vi "FPGA_DATA.vi"() -> ()   [LabVIEW 2019]
uses:
  <vilib>/LabVIEW Targets/FPGA/RIO/nicrio_985x_controls.llb/CAN_IO_Frame Cluster.ctl
  <vilib>/LabVIEW Targets/FPGA/RIO/nicrio_985x_controls.llb/CAN_IO_Frame Type.ctl
  <vilib>/rvi/Emulation/niFpgaGetClockAttributes.vi
  <vilib>/rvi/Emulation/niFpgaSctlEmulationGetInTimedLoop.vi
  <vilib>/rvi/Emulation/niFpgaEmulationReportErrorSimple.vi
  <vilib>/rvi/eio/common/nirviEmuTemplateMethod_errors.vi
  <vilib>/rvi/Emulation/niFpgaCriticalErrorInLSC.vi
  <vilib>/eio/EIONode/EIONode.xnode
panel:
  in  "DIO1":bool
  in  "CAN1 write":T1={"배열[0]"={"timestamp high"=0, "timestamp low"=0, "identifier"=0, "type"=enum."Data Frame", "info A"=0, "info B"=0, "data length"=0, "data"=[0, 0, 0, 0, 0, 0, 0, 0]}, "배열[1]"={"timestamp high"=0, "timestamp low"=0, "identifier"=0, "type"=enum."Data Frame", "info A"=0, "info B"=0, "data length"=0, "data"=[0, 0, 0, 0, 0, 0, 0, 0]}, "배열[2]"={"timestamp high"=0, "timestamp low"=0, "identifier"=0, "type"=enum."Data Frame", "info A"=0, "info B"=0, "data length"=0, "data"=[0, 0, 0, 0, 0, 0, 0, 0]}, "배열[3]"={"timestamp high"=0, "timestamp low"=0, "identifier"=0, "type"=enum."Data Frame", "info A"=0, "info B"=0, "data length"=0, "data"=[0, 0, 0, 0, 0, 0, 0, 0]}, "배열[4]"={"timestamp high"=0, "timestamp low"=0, "identifier"=0, "type"=enum."Data Frame", "info A"=0, "info B"=0, "data length"=0, "data"=[0, 0, 0, 0, 0, 0, 0, 0]}}
  out "L_force":sgl
  out "R_force":sgl
  out "CAN1 read":T2={"배열 2[0]"={"timestamp high"=0, "timestamp low"=0, "identifier"=0, "type"=enum."Data Frame", "info A"=0, "info B"=0, "data length"=0, "data"=[0, 0, 0, 0, 0, 0, 0, 0]}}
  in  "Write_que":bool
  out "Mod1/CAN1":T3={"timestamp high"=0, "timestamp low"=0, "identifier"=0, "type"=enum."Data Frame", "info A"=0, "info B"=0, "data length"=0, "data"=[0, 0, 0, 0, 0, 0, 0, 0]} {"identifier" format="%x"; "timestamp high" format="%08x"; "timestamp low" format="%08x"; "data" format="%.0x"}
  in  "D2":bool
  out "IMUS":sgl[](array[numeric])
  out "Mod1/CAN0":T3={"timestamp high"=0, "timestamp low"=0, "identifier"=0, "type"=enum."Data Frame", "info A"=0, "info B"=0, "data length"=0, "data"=[0, 0, 0, 0, 0, 0, 0, 0]} {"identifier" format="%x"; "timestamp high" format="%08x"; "timestamp low" format="%08x"; "data" format="%.0x"}
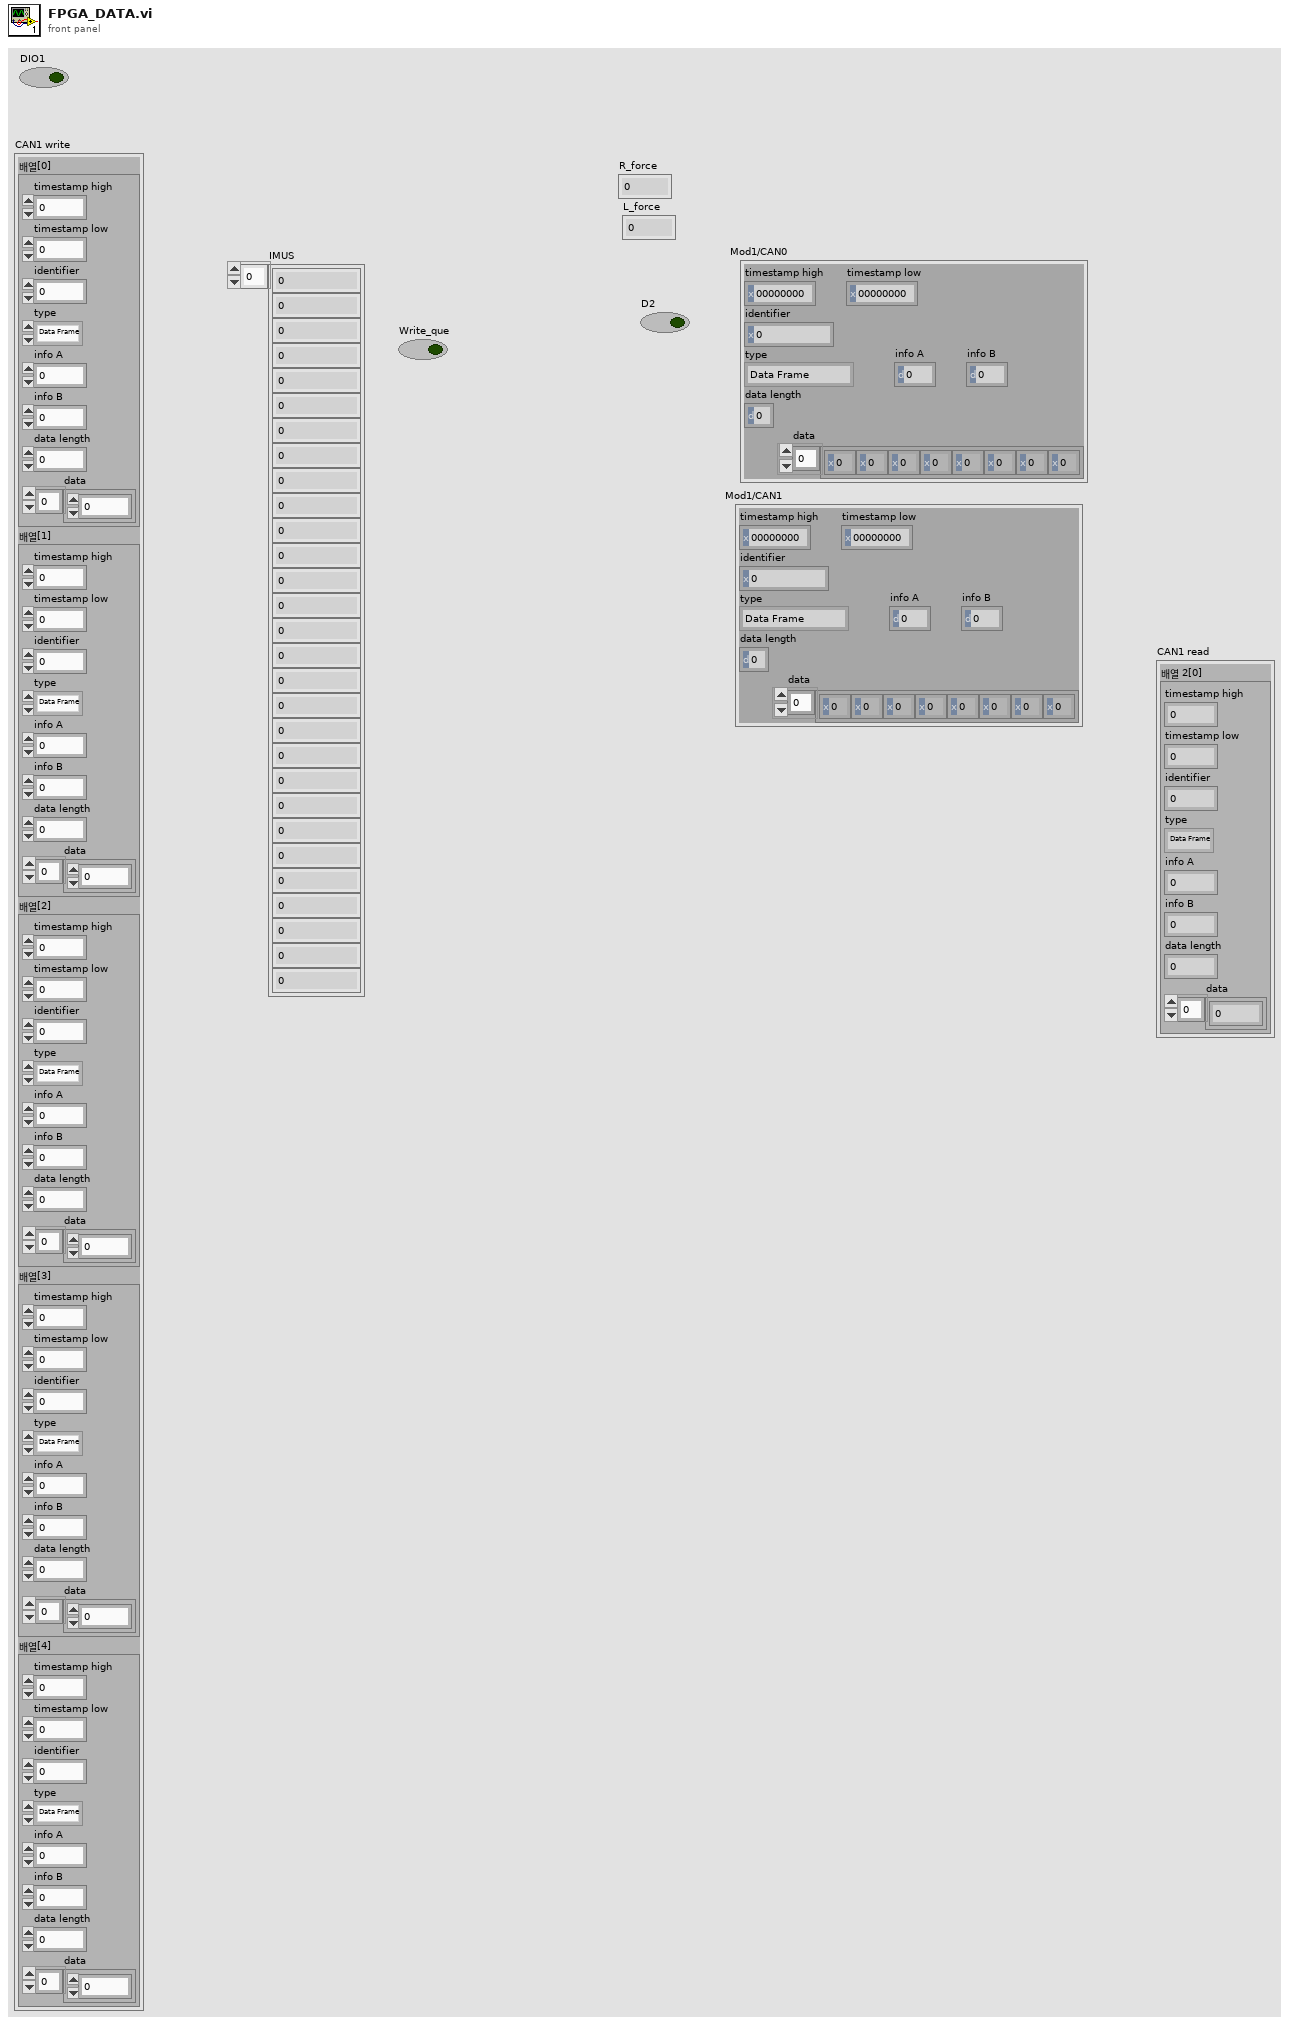
[diagram p1: front panel]
types:
  T1 = cluster{"배열[0]":cluster{"timestamp high":u32, "timestamp low":u32, "identifier":u32, "type":enum8{"Data Frame", "Remote Frame", "(reserved)", "(reserved) ", "(reserved)  ", "(reserved)   ", "Bus Error", "Transceiver Fault"}, "info A":u8, "info B":u8, "data length":u8, "data":u8[]}, "배열[1]":cluster{"timestamp high":u32, "timestamp low":u32, "identifier":u32, "type":enum8{"Data Frame", "Remote Frame", "(reserved)", "(reserved) ", "(reserved)  ", "(reserved)   ", "Bus Error", "Transceiver Fault"}, "info A":u8, "info B":u8, "data length":u8, "data":u8[]}, "배열[2]":cluster{"timestamp high":u32, "timestamp low":u32, "identifier":u32, "type":enum8{"Data Frame", "Remote Frame", "(reserved)", "(reserved) ", "(reserved)  ", "(reserved)   ", "Bus Error", "Transceiver Fault"}, "info A":u8, "info B":u8, "data length":u8, "data":u8[]}, "배열[3]":cluster{"timestamp high":u32, "timestamp low":u32, "identifier":u32, "type":enum8{"Data Frame", "Remote Frame", "(reserved)", "(reserved) ", "(reserved)  ", "(reserved)   ", "Bus Error", "Transceiver Fault"}, "info A":u8, "info B":u8, "data length":u8, "data":u8[]}, "배열[4]":cluster{"timestamp high":u32, "timestamp low":u32, "identifier":u32, "type":enum8{"Data Frame", "Remote Frame", "(reserved)", "(reserved) ", "(reserved)  ", "(reserved)   ", "Bus Error", "Transceiver Fault"}, "info A":u8, "info B":u8, "data length":u8, "data":u8[]}}
  T2 = cluster{"배열 2[0]":cluster{"timestamp high":u32, "timestamp low":u32, "identifier":u32, "type":enum8{"Data Frame", "Remote Frame", "(reserved)", "(reserved) ", "(reserved)  ", "(reserved)   ", "Bus Error", "Transceiver Fault"}, "info A":u8, "info B":u8, "data length":u8, "data":u8[]}}
  T3 = typedef "CAN_IO_Frame Cluster.ctl" = cluster{"timestamp high":u32, "timestamp low":u32, "identifier":u32, "type":T4, "info A":u8, "info B":u8, "data length":u8, "data":u8[]}
  T4 = typedef "CAN_IO_Frame Type.ctl" = enum8{"Data Frame", "Remote Frame", "(reserved)", "(reserved) ", "(reserved)  ", "(reserved)   ", "Bus Error", "Transceiver Fault"}
  T5 = cluster{"timestamp high":u32, "timestamp low":u32, "identifier":u32, "type":enum8{"Data Frame", "Remote Frame", "(reserved)", "(reserved) ", "(reserved)  ", "(reserved)   ", "Bus Error", "Transceiver Fault"}, "info A":u8, "info B":u8, "data length":u8, "data":u8[]}[]
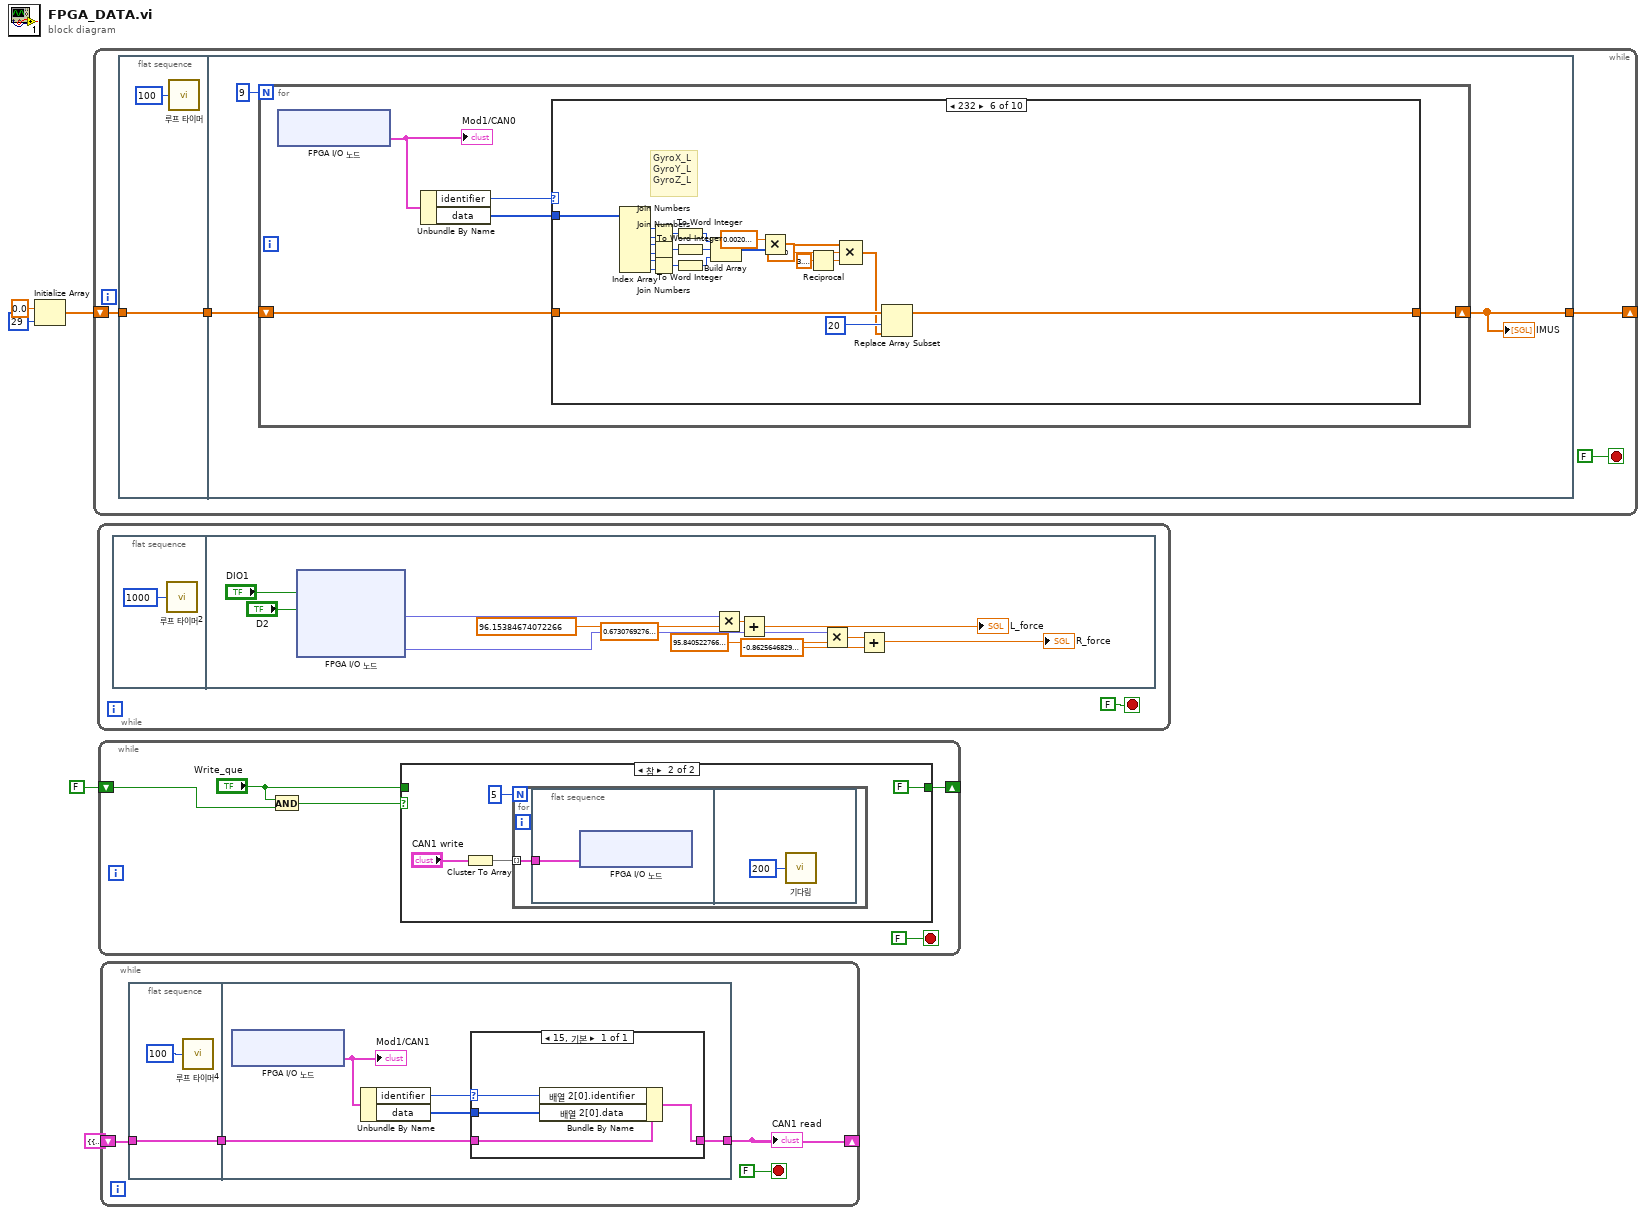
[diagram p0: block diagram]
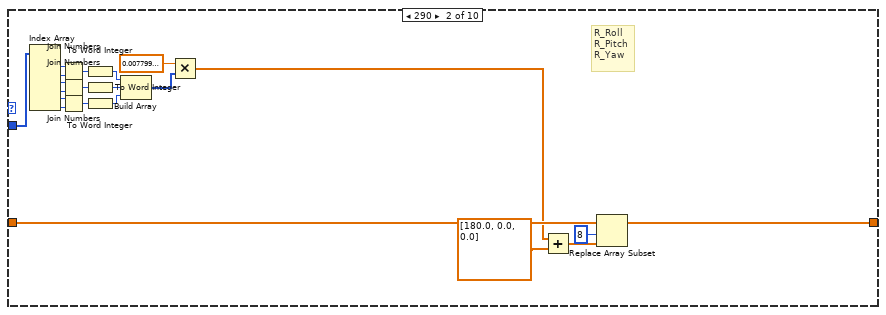
[diagram p3: hidden frame]
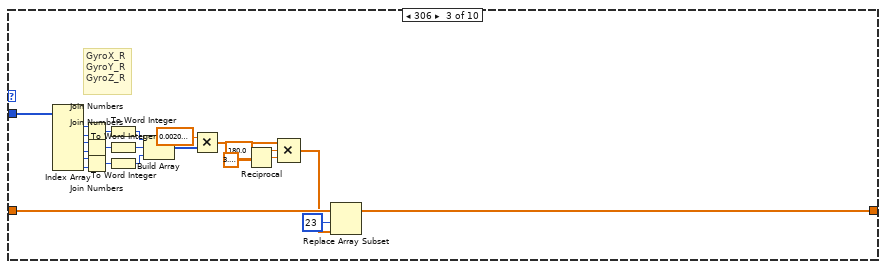
[diagram p4: hidden frame]
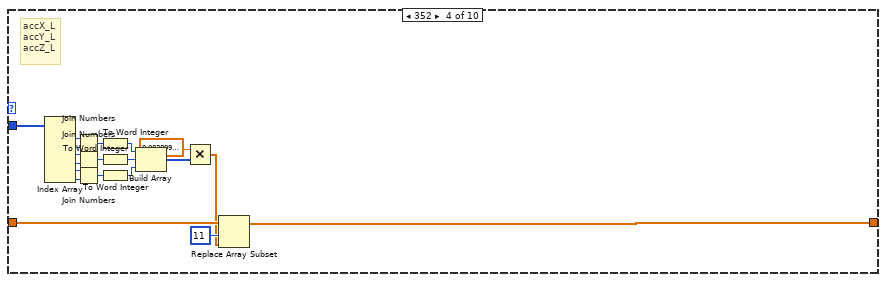
[diagram p5: hidden frame]
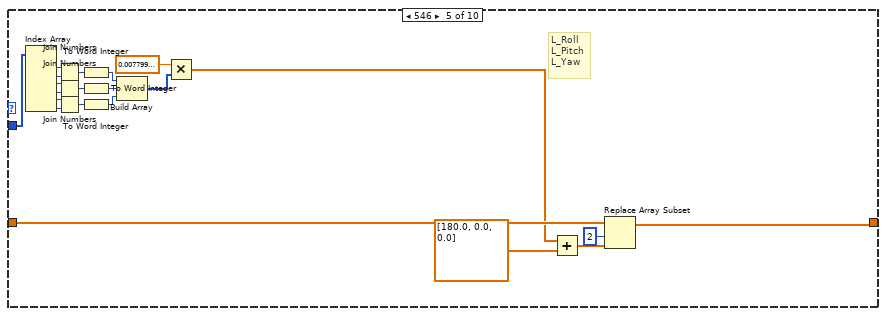
[diagram p6: hidden frame]
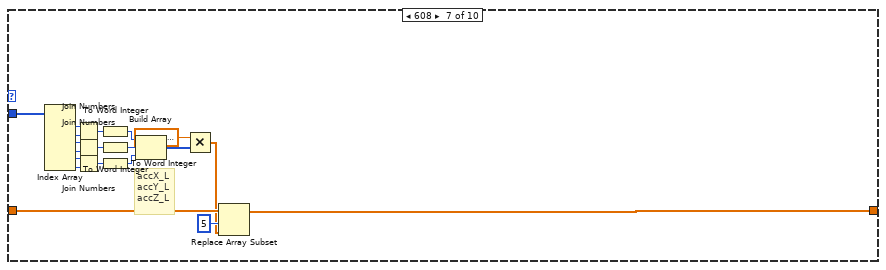
[diagram p7: hidden frame]
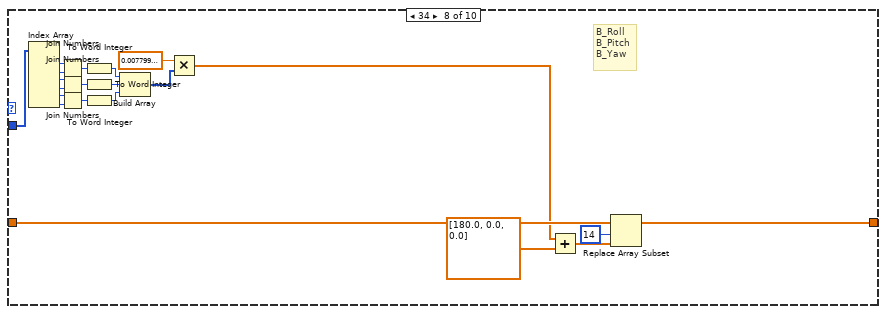
[diagram p8: hidden frame]
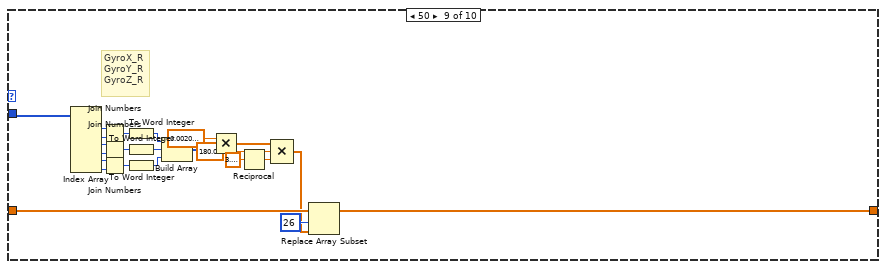
[diagram p9: hidden frame]
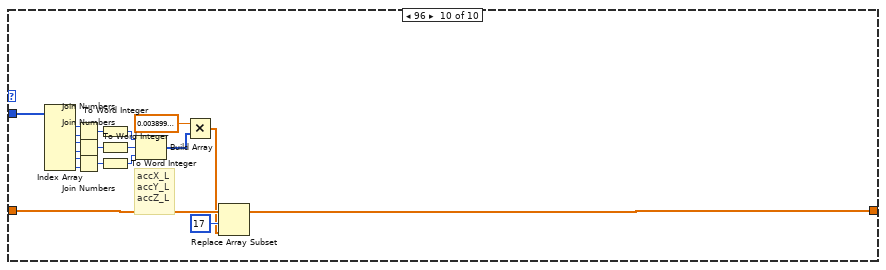
[diagram p10: hidden frame]
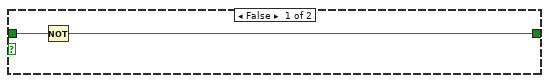
[diagram p11: hidden frame]
diagram:
  n1 = Initialize Array(sgl 0.0 ("timeout (0 s)"), 29 ("차원 크기")) -> (w3:sgl[])
  n2 = while {
    shift-right: [w8] -> _
    shift-left: w3 -> [w7]
    stop <- FALSE stop-if-true
    n3 = flat-sequence {
      tunnel: w7 -> [w10]
      tunnel: [w10] -> w6
      tunnel: [w12] -> w8
      tunnel: w6 -> [w14]
      frame #0 {
        n4 = call "루프 타이머"("Count(mSec)"=u32 100) -> ()  [unwired: 1 out]
      }
      frame #1 {
        n5 = for {
          N: 9 -> [_]
          shift-right: [w16] -> w12
          shift-left: w14 -> [w15]
          n6 = xnode "FPGA I/O 노드"() -> ("Mod1/CAN0"=w17:T3)  [unwired: 1 in, 1 out]
          "Mod1/CAN0" <- w17
          n7 = Unbundle By Name(w17) -> ("identifier"=w19:u32, "data"=w18:u8[])
          n8 = case shown="232" w19 {
            tunnel: w18 -> [_ w41 w49 w77 w104 w112 w140 w167 w175 w203]
            tunnel: w15 -> [w20 w40 w48 w76 w86 w111 w139 w166 w174 w202]
            tunnel: [w20 w23 w47 w74 w85 w110 w137 w148 w173 w200] -> w16
            frame 0, Default {
            }
            frame 290 {
              # "R_Roll\nR_Pitch\nR_Yaw"
              n9 = Index Array(array=w41) -> (element #1=w34:u8, element #2=w35:u8, element #3=w36:u8, element #4=w37:u8, element #5=w38:u8, element #6=w39:u8)  [unwired: 6 in]
              n10 = Join Numbers(hi=w34, lo=w35) -> ((hi.lo)=w32:u16)
              n11 = Join Numbers(hi=w36, lo=w37) -> ((hi.lo)=w30:u16)
              n12 = Join Numbers(hi=w38, lo=w39) -> ((hi.lo)=w31:u16)
              n13 = To Word Integer(number=w32) -> (16bit integer=w28:i16)
              n14 = To Word Integer(number=w30) -> (16bit integer=w27:i16)
              n15 = To Word Integer(number=w31) -> (16bit integer=w26:i16)
              n16 = Build Array(w28, w27, w26) -> (w25:i16[])
              n17 = Multiply ("곱하기")(x=sgl 0.0078, y=w25) -> (x*y=w21:sgl[])
              n18 = Add(x=w21, y=sgl[] [180.0, 0.0, 0.0]) -> (x+y=w22:sgl[])
              n19 = Replace Array Subset(array=w40, new element=w22, index=8 ("인덱스")) -> (w23:sgl[])
            }
            frame 306 {
              # "GyroX_R\nGyroY_R\nGyroZ_R"
              n20 = Index Array(array=w49) -> (element #1=w59:u8, element #2=w60:u8, element #3=w61:u8, element #4=w62:u8, element #5=w63:u8, element #6=w64:u8)  [unwired: 6 in]
              n21 = Join Numbers(hi=w59, lo=w60) -> ((hi.lo)=w57:u16)
              n22 = Join Numbers(hi=w61, lo=w62) -> ((hi.lo)=w55:u16)
              n23 = Join Numbers(hi=w63, lo=w64) -> ((hi.lo)=w56:u16)
              n24 = To Word Integer(number=w57) -> (16bit integer=w53:i16)
              n25 = To Word Integer(number=w55) -> (16bit integer=w52:i16)
              n26 = To Word Integer(number=w56) -> (16bit integer=w51:i16)
              n27 = Build Array(w53, w52, w51) -> (w50:i16[])
              n28 = Multiply ("곱하기")(x=sgl 0.002, y=w50) -> (x*y=w46:sgl[])
              n29 = Reciprocal(x=sgl 3.1415927) -> (1/x=w45:sgl)
              n30 = Compound Arithmetic op=MULTIPLY(w46, sgl 180.0 ("값"), w45) -> (w44:sgl[])
              n31 = Replace Array Subset(array=w48, new element=w44, index=23 ("인덱스")) -> (w47:sgl[])
            }
            frame 352 {
              # "accX_L\naccY_L\naccZ_L"
              n32 = Index Array(array=w77) -> (element #1=w78:u8, element #2=w79:u8, element #3=w80:u8, element #4=w81:u8, element #5=w82:u8, element #6=w83:u8)  [unwired: 6 in]
              n33 = Join Numbers(hi=w78, lo=w79) -> ((hi.lo)=w73:u16)
              n34 = Join Numbers(hi=w80, lo=w81) -> ((hi.lo)=w71:u16)
              n35 = Join Numbers(hi=w82, lo=w83) -> ((hi.lo)=w72:u16)
              n36 = To Word Integer(number=w73) -> (16bit integer=w69:i16)
              n37 = To Word Integer(number=w71) -> (16bit integer=w68:i16)
              n38 = To Word Integer(number=w72) -> (16bit integer=w67:i16)
              n39 = Build Array(w69, w68, w67) -> (w66:i16[])
              n40 = Multiply ("곱하기")(x=sgl 0.0039, y=w66) -> (x*y=w65:sgl[])
              n41 = Replace Array Subset(array=w76, new element=w65, index=11 ("인덱스")) -> (w74:sgl[])
            }
            frame 546 {
              # "L_Roll\nL_Pitch\nL_Yaw"
              n42 = Index Array(array=w104) -> (element #1=w98:u8, element #2=w99:u8, element #3=w100:u8, element #4=w101:u8, element #5=w102:u8, element #6=w103:u8)  [unwired: 6 in]
              n43 = Join Numbers(hi=w98, lo=w99) -> ((hi.lo)=w95:u16)
              n44 = Join Numbers(hi=w100, lo=w101) -> ((hi.lo)=w93:u16)
              n45 = Join Numbers(hi=w102, lo=w103) -> ((hi.lo)=w94:u16)
              n46 = To Word Integer(number=w95) -> (16bit integer=w91:i16)
              n47 = To Word Integer(number=w93) -> (16bit integer=w90:i16)
              n48 = To Word Integer(number=w94) -> (16bit integer=w89:i16)
              n49 = Build Array(w91, w90, w89) -> (w88:i16[])
              n50 = Multiply ("곱하기")(x=sgl 0.0078, y=w88) -> (x*y=w84:sgl[])
              n51 = Add(x=w84, y=sgl[] [180.0, 0.0, 0.0]) -> (x+y=w96:sgl[])
              n52 = Replace Array Subset(array=w86, new element=w96, index=2 ("인덱스")) -> (w85:sgl[])
            }
            frame 562 {
              # "GyroX_L\nGyroY_L\nGyroZ_L"
              n53 = Index Array(array=w112) -> (element #1=w120:u8, element #2=w119:u8, element #3=w118:u8, element #4=w117:u8, element #5=w116:u8, element #6=w115:u8)  [unwired: 6 in]
              n54 = Join Numbers(hi=w120, lo=w119) -> ((hi.lo)=w121:u16)
              n55 = Join Numbers(hi=w118, lo=w117) -> ((hi.lo)=w123:u16)
              n56 = Join Numbers(hi=w116, lo=w115) -> ((hi.lo)=w122:u16)
              n57 = To Word Integer(number=w121) -> (16bit integer=w124:i16)
              n58 = To Word Integer(number=w123) -> (16bit integer=w125:i16)
              n59 = To Word Integer(number=w122) -> (16bit integer=w126:i16)
              n60 = Build Array(w124, w125, w126) -> (w127:i16[])
              n61 = Multiply ("곱하기")(x=sgl 0.002, y=w127) -> (x*y=w108:sgl[])
              n62 = Reciprocal(x=sgl 3.1415927) -> (1/x=w109:sgl)
              n63 = Compound Arithmetic op=MULTIPLY(w108, sgl 180.0 ("값"), w109) -> (w107:sgl[])
              n64 = Replace Array Subset(array=w111, new element=w107, index=20 ("인덱스")) -> (w110:sgl[])
            }
            frame 608 {
              # "accX_L\naccY_L\naccZ_L"
              n65 = Index Array(array=w140) -> (element #1=w141:u8, element #2=w142:u8, element #3=w143:u8, element #4=w144:u8, element #5=w145:u8, element #6=w146:u8)  [unwired: 6 in]
              n66 = Join Numbers(hi=w141, lo=w142) -> ((hi.lo)=w136:u16)
              n67 = Join Numbers(hi=w143, lo=w144) -> ((hi.lo)=w134:u16)
              n68 = Join Numbers(hi=w145, lo=w146) -> ((hi.lo)=w135:u16)
              n69 = To Word Integer(number=w136) -> (16bit integer=w132:i16)
              n70 = To Word Integer(number=w134) -> (16bit integer=w131:i16)
              n71 = To Word Integer(number=w135) -> (16bit integer=w130:i16)
              n72 = Build Array(w132, w131, w130) -> (w129:i16[])
              n73 = Multiply ("곱하기")(x=sgl 0.0039, y=w129) -> (x*y=w128:sgl[])
              n74 = Replace Array Subset(array=w139, new element=w128, index=5 ("인덱스")) -> (w137:sgl[])
            }
            frame 34 {
              # "B_Roll\nB_Pitch\nB_Yaw"
              n75 = Index Array(array=w167) -> (element #1=w160:u8, element #2=w161:u8, element #3=w162:u8, element #4=w163:u8, element #5=w164:u8, element #6=w165:u8)  [unwired: 6 in]
              n76 = Join Numbers(hi=w160, lo=w161) -> ((hi.lo)=w157:u16)
              n77 = Join Numbers(hi=w162, lo=w163) -> ((hi.lo)=w155:u16)
              n78 = Join Numbers(hi=w164, lo=w165) -> ((hi.lo)=w156:u16)
              n79 = To Word Integer(number=w157) -> (16bit integer=w153:i16)
              n80 = To Word Integer(number=w155) -> (16bit integer=w152:i16)
              n81 = To Word Integer(number=w156) -> (16bit integer=w151:i16)
              n82 = Build Array(w153, w152, w151) -> (w150:i16[])
              n83 = Multiply ("곱하기")(x=sgl 0.0078, y=w150) -> (x*y=w147:sgl[])
              n84 = Add(x=w147, y=sgl[] [180.0, 0.0, 0.0]) -> (x+y=w158:sgl[])
              n85 = Replace Array Subset(array=w166, new element=w158, index=14 ("인덱스")) -> (w148:sgl[])
            }
            frame 50 {
              # "GyroX_R\nGyroY_R\nGyroZ_R"
              n86 = Index Array(array=w175) -> (element #1=w185:u8, element #2=w186:u8, element #3=w187:u8, element #4=w188:u8, element #5=w189:u8, element #6=w190:u8)  [unwired: 6 in]
              n87 = Join Numbers(hi=w185, lo=w186) -> ((hi.lo)=w183:u16)
              n88 = Join Numbers(hi=w187, lo=w188) -> ((hi.lo)=w181:u16)
              n89 = Join Numbers(hi=w189, lo=w190) -> ((hi.lo)=w182:u16)
              n90 = To Word Integer(number=w183) -> (16bit integer=w179:i16)
              n91 = To Word Integer(number=w181) -> (16bit integer=w178:i16)
              n92 = To Word Integer(number=w182) -> (16bit integer=w177:i16)
              n93 = Build Array(w179, w178, w177) -> (w176:i16[])
              n94 = Multiply ("곱하기")(x=sgl 0.002, y=w176) -> (x*y=w171:sgl[])
              n95 = Reciprocal(x=sgl 3.1415927) -> (1/x=w172:sgl)
              n96 = Compound Arithmetic op=MULTIPLY(w171, sgl 180.0 ("값"), w172) -> (w170:sgl[])
              n97 = Replace Array Subset(array=w174, new element=w170, index=26 ("인덱스")) -> (w173:sgl[])
            }
            frame 96 {
              # "accX_L\naccY_L\naccZ_L"
              n98 = Index Array(array=w203) -> (element #1=w204:u8, element #2=w205:u8, element #3=w206:u8, element #4=w207:u8, element #5=w208:u8, element #6=w209:u8)  [unwired: 6 in]
              n99 = Join Numbers(hi=w204, lo=w205) -> ((hi.lo)=w199:u16)
              n100 = Join Numbers(hi=w206, lo=w207) -> ((hi.lo)=w197:u16)
              n101 = Join Numbers(hi=w208, lo=w209) -> ((hi.lo)=w198:u16)
              n102 = To Word Integer(number=w199) -> (16bit integer=w195:i16)
              n103 = To Word Integer(number=w197) -> (16bit integer=w194:i16)
              n104 = To Word Integer(number=w198) -> (16bit integer=w193:i16)
              n105 = Build Array(w195, w194, w193) -> (w192:i16[])
              n106 = Multiply ("곱하기")(x=sgl 0.0039, y=w192) -> (x*y=w191:sgl[])
              n107 = Replace Array Subset(array=w202, new element=w191, index=17 ("인덱스")) -> (w200:sgl[])
            }
          }
        }
        "IMUS" <- w12
      }
    }
  }
  n108 = while {
    stop <- FALSE stop-if-true
    n109 = flat-sequence {
      frame #0 {
        n110 = call "루프 타이머2"("Count(uSec)"=u32 1000 ("Count(mSec)")) -> ()  [unwired: 1 out]
      }
      frame #1 {
        n111 = xnode "FPGA I/O 노드"("Mod3/DIO1"="DIO1", "Mod3/DIO0"="D2") -> ("Mod3/AI1"=w221:fxp<+,18,3>, "Mod3/AI2"=w220:fxp<+,18,3>)  [unwired: 4 in, 4 out]
        n112 = Multiply ("곱하기")(x=w221, y=sgl 96.15385) -> (x*y=w219:sgl)
        n113 = Add(x=w219, y=sgl 0.6730769) -> (x+y=→"L_force":sgl)
        n114 = Multiply ("곱하기")(x=w220, y=sgl 95.84052) -> (x*y=w217:sgl)
        n115 = Add(x=w217, y=sgl -0.8625647) -> (x+y=→"R_force":sgl)
      }
    }
  }
  n116 = while {
    shift-right: [w225] -> _
    shift-left: FALSE -> [w226]
    stop <- FALSE stop-if-true
    n117 = And(x="Write_que", y=w226) -> (x .and. y?=w227:bool)
    n118 = case shown="참" w227 {
      tunnel: [w229 FALSE] -> w225
      tunnel: "Write_que" -> [w230 _]
      frame False {
        n119 = Not(x=w230) -> (.not. x?=w229:bool)
      }
      frame True {
        n120 = Cluster To Array(cluster="CAN1 write") -> (array=w233:T5)
        n121 = for "For 루프" {
          N: 5 -> [_]
          tunnel: w233 -> [w235] mode=indexing
          n122 = flat-sequence {
            tunnel: w235 -> [w236]
            frame #0 {
              n123 = xnode "FPGA I/O 노드"("Mod1/CAN1"=w236) -> ()  [unwired: 1 in, 1 out]
            }
            frame #1 {
              n124 = call "기다림"("Count(uSec)"=u32 200 ("Count(mSec)")) -> ()  [unwired: 1 out]
            }
          }
        }
      }
    }
  }
  n125 = while {
    shift-right: [w240] -> _
    shift-left: T2 {"배열 2[0]"={"timestamp high"=0, "timestamp low"=0, "identifier"=0, "type"=enum."Data Frame", "info A"=0, "info B"=0, "data length"=0, "data"=[0, 0, 0, 0, 0, 0, 0, 0]}} ("클러스터") -> [w239]
    stop <- FALSE stop-if-true
    n126 = flat-sequence {
      tunnel: [w242] -> w241
      tunnel: w239 -> [w242]
      tunnel: w241 -> [w248]
      tunnel: [w247] -> w240
      frame #0 {
        n127 = call "루프 타이머4"("Count(uSec)"=u32 100 ("Count(mSec)")) -> ()  [unwired: 1 out]
      }
      frame #1 {
        n128 = xnode "FPGA I/O 노드"() -> ("Mod1/CAN1"=w246:T3)  [unwired: 1 in, 1 out]
        "Mod1/CAN1" <- w246
        n129 = Unbundle By Name(w246) -> ("identifier"=w245:u32, "data"=w244:u8[])
        n130 = case shown="15, 기본" w245 {
          selector: w245 -> [w249]
          tunnel: w244 -> [w251]
          tunnel: w248 -> [w252]
          tunnel: [w250] -> w247
          frame 15, Default {
            n131 = Bundle By Name(cluster=w252, "배열 2[0].identifier"=w249, "배열 2[0].data"=w251) -> (w250:T2)
          }
        }
      }
    }
    "CAN1 read" <- w240
  }
